vi "ACTOR_VI_NAMES_TEMPLATE_ONLY.vi"(8 "error in (no error)":errorcluster, 11 "Actor-Class Item":T1) -> (0 "error out":errorcluster, 3 "Name":string="Run.vi")   [LabVIEW 2018, in "Templates.lvlib" / "Actor.lvclass"]
uses:
  Actor.lvclass
  Actor Class Items.ctl
  Create Message-Enqueuer References.vi
  Destroy Message-Enqueuer References.vi
  Message-Enqueuer References.ctl
  Messages.ctl
  Run.vi
  Templates.lvlib
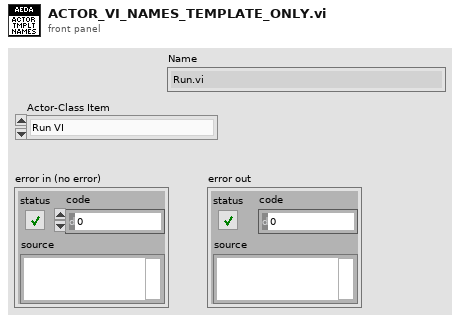
[diagram p1: front panel]
types:
  T1 = typedef "Templates.lvlib/Actor Class Items.ctl" = enum16{"Run VI", "Create Enqueuers VI", "Destroy Enqueuers VI", "Enqueuers Control", "Messages Control"}
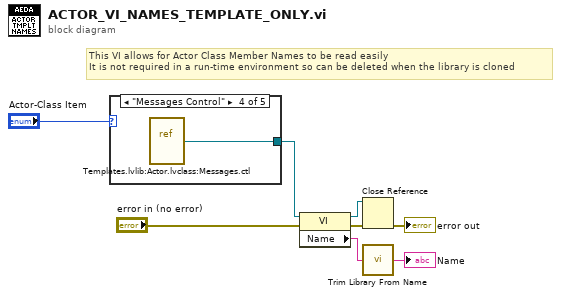
[diagram p0: block diagram]
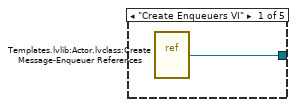
[diagram p2: hidden frame]
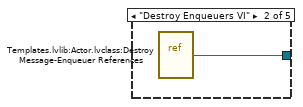
[diagram p3: hidden frame]
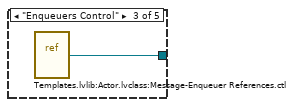
[diagram p4: hidden frame]
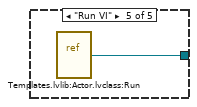
[diagram p5: hidden frame]
diagram:
  # "This VI allows for Actor Class Member Names to be read easily\nIt is not required in a run-time environment so can be deleted when the library is cloned"
  n1 = case shown="\"Messages Control\"" "Actor-Class Item" {
    tunnel: [w9 w10 w11 w12 w13] -> w4
    frame "Create Enqueuers VI" {
      n2 = vi-ref "Templates.lvlib:Actor.lvclass:Create Message-Enqueuer References.vi"() -> (w9:refnum<vi>)
    }
    frame "Destroy Enqueuers VI" {
      n3 = vi-ref "Templates.lvlib:Actor.lvclass:Destroy Message-Enqueuer References.vi"() -> (w10:refnum<vi>)
    }
    frame "Enqueuers Control" {
      n4 = vi-ref "Templates.lvlib:Actor.lvclass:Message-Enqueuer References.ctl"() -> (w11:refnum<vi>)
    }
    frame "Messages Control" {
      n5 = vi-ref "Templates.lvlib:Actor.lvclass:Messages.ctl"() -> (w12:refnum<vi>)
    }
    frame "Run VI" {
      n6 = vi-ref "Templates.lvlib:Actor.lvclass:Run.vi"() -> (w13:refnum<vi>)
    }
  }
  n7 = property class="VI"(reference=w4, error in="error in (no error)") -> (reference out=w2:refnum<vi>, error out=w3:errorcluster, "Name"=w1:string)
  n8 = Close Reference(reference=w2, error in (no error)=w3) -> (error out=→"error out":errorcluster)
  n9 = call "Trim Library From Name.vi"("Name in"=w1) -> ("Name out"=→"Name":string)
